vi "DetectChange.vi"(11 "Value":i32) -> (3 "Changed":bool)   [LabVIEW 2023]
doc: "Returns true if the value changed"
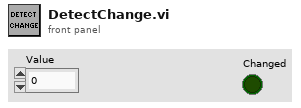
[diagram p1: front panel]
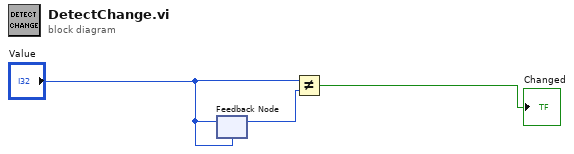
[diagram p0: block diagram]
diagram:
  n1 = feedback-in #1("Value") -> ()
  n2 = feedback #1("Value") -> (w3:i32)
  n3 = Not Equal?(x="Value", y=w3) -> (x != y?=→"Changed":bool)
